vi "set_visaResource.vi"(0 "HGF_VISADevice":refnum<class "HGF_VISADevice.lvclass">, 2 "visaResource":refnum<visa-resource-name>, 5 "error in (no error)":errorcluster) -> (14 "dup HGF_VISADevice":refnum<class "HGF_VISADevice.lvclass">, 19 "error out":errorcluster)   [LabVIEW 2014, in "HGF_DeviceBaseClasses.lvlib" / "HGF_VISADevice.lvclass"]
doc: "Modify the VISA Resource from the instrument's initialize.vi."
uses:
  HGF_VISADevice.lvclass
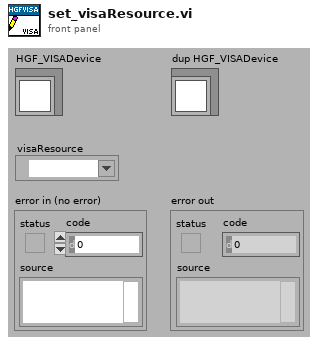
[diagram p1: front panel]
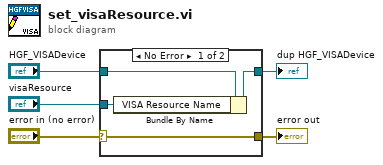
[diagram p0: block diagram]
diagram:
  n1 = case shown="No Error" "error in (no error)" {
    selector: "error in (no error)" -> [w9 w10]
    tunnel: [w9 w10] -> w4
    tunnel: [w7 w11] -> w2
    tunnel: "HGF_VISADevice" -> [w8 w11]
    tunnel: "visaResource" -> [w6 _]
    frame No Error {
      n2 = Bundle By Name(cluster=w8, "VISA Resource Name"=w6) -> (w7:refnum<class "HGF_VISADevice.lvclass">)
    }
    frame Error {
    }
  }
  "error out" <- w4
  "dup HGF_VISADevice" <- w2
